vi "Read Gain.vi"(8 "error in (no error)":errorcluster, 11 "KH7008 in":refnum<class "Instrument.KH7008.lvclass">) -> (0 "error out":errorcluster, 2 "Gain":dbl[](array[numeric]), 3 "KH7008 out":refnum<class "Instrument.KH7008.lvclass">)   [LabVIEW 2019, in "Instrument.KH7008.lvclass"]
uses:
  <userlib>/LevyLab/Krohn Hite 7008/Instrument.KH7008.lvclass
  <userlib>/LevyLab/Krohn Hite 7008/Instrument.KH7008.lvclass/Instrument.KH7008.ctl
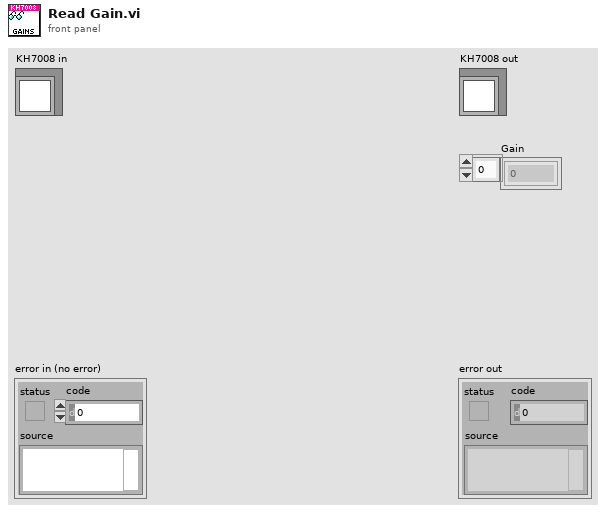
[diagram p1: front panel]
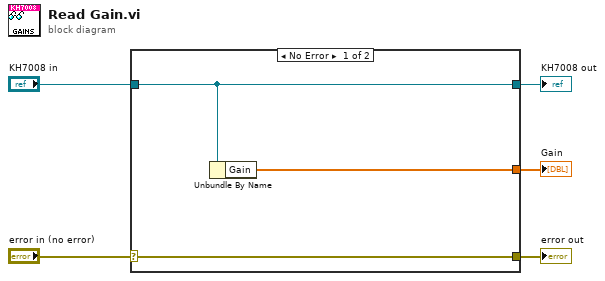
[diagram p0: block diagram]
diagram:
  n1 = case shown="No Error" "error in (no error)" {
    selector: "error in (no error)" -> [w8 w9]
    tunnel: [w8 w9] -> w4
    tunnel: [w7 w10] -> w2
    tunnel: "KH7008 in" -> [w7 w10]
    tunnel: [w6 _] -> w1
    frame No Error {
      n2 = Unbundle By Name(w7) -> ("Gain"=w6:dbl[])
    }
    frame Error {
    }
  }
  "error out" <- w4
  "KH7008 out" <- w2
  "Gain" <- w1
